vi "Get Selected Text Format.vi"(8 "Error In":errorcluster, 11 "Text Formatting in":T5 {"Font Size" min=6.0 step=1.0}) -> (0 "Error Out":errorcluster, 3 "Text Formatting":T4={"Font"=0, "Text Color"=enum."Unchanged", "Background Color"=enum."Unchanged", "Style"=enum."Regular", "Font Size"=6.0, "Alignment"=enum."Left"} {"Font Size" min=6.0 step=1.0; "Font" items=["Adobe Devanagari", "Agency FB", "Algerian", "Arial", "Arial Black", "Arial Narrow", "Arial Rounded MT Bold", "Bahnschrift", "Bahnschrift Condensed", "Bahnschrift Light", "Bahnschrift Light Condensed", "Bahnschrift Light SemiCondensed", "Bahnschrift SemiBold", "Bahnschrift SemiBold Condensed", "Bahnschrift SemiBold SemiConden", "Bahnschrift SemiCondensed", "Bahnschrift SemiLight", "Bahnschrift SemiLight Condensed", "Bahnschrift SemiLight SemiConde", "Barlow Condensed", "Barlow Condensed Black", "Barlow Condensed ExtraBold", "Barlow Condensed ExtraLight", "Barlow Condensed Light", "Barlow Condensed Medium", "Barlow Condensed SemiBold", "Barlow Condensed Thin", "Baskerville Old Face", "Bauhaus 93", "Bell MT", "Berlin Sans FB", "Berlin Sans FB Demi", "Bernard MT Condensed", "Blackadder ITC", "Bodoni MT", "Bodoni MT Black", "Bodoni MT Condensed", "Bodoni MT Poster Compressed", "Book Antiqua", "Bookman Old Style", "Bookshelf Symbol 7", "Bradley Hand ITC", "Britannic Bold", "Broadway", "Brush Script MT", "Calibri", "Calibri Light", "Californian FB", "Calisto MT", "Cambria", "Cambria Math", "Candara", "Candara Light", "Cascadia Code", "Cascadia Code ExtraLight", "Cascadia Code Light", "Cascadia Code SemiBold", "Cascadia Code SemiLight", "Cascadia Mono", "Cascadia Mono ExtraLight", "Cascadia Mono Light", "Cascadia Mono SemiBold", "Cascadia Mono SemiLight", "Castellar", "Caveat", "Centaur", "Century", "Century Gothic", "Century Schoolbook", "Chiller", "Colonna MT", "Comic Sans MS", "Consolas", "Constantia", "Cooper Black", "Copperplate Gothic Bold", "Copperplate Gothic Light", "Corbel", "Corbel Light", "Cormorant Infant", "Cormorant Infant Light", "Cormorant Infant Medium", "Cormorant Infant SemiBold", "Courier New", "Curlz MT", "Dosis", "Dubai", "Dubai Light", "Dubai Medium", "Ebrima", "Edwardian Script ITC", "Elephant", "Engravers MT", "Eras Bold ITC", "Eras Demi ITC", "Eras Light ITC", "Eras Medium ITC", "Euclid", "Euclid Extra", "Euclid Fraktur", "Euclid Math One", "Euclid Math Two", "Euclid Symbol", "Felix Titling", "Fences", "Footlight MT Light", "Forte", "Franklin Gothic Book", "Franklin Gothic Demi", "Franklin Gothic Demi Cond", "Franklin Gothic Heavy", "Franklin Gothic Medium", "Franklin Gothic Medium Cond", "Freestyle Script", "French Script MT", "Gabriola", "Gadugi", "Garamond", "Georgia", "Gigi", "Gill Sans MT", "Gill Sans MT Condensed", "Gill Sans MT Ext Condensed Bold", "Gill Sans Ultra Bold", "Gill Sans Ultra Bold Condensed", "Gloucester MT Extra Condensed", "Goudy Old Style", "Goudy Stout", "Haettenschweiler", "Harlow Solid Italic", "Harrington", "High Tower Text", "HoloLens MDL2 Assets", "HYSWLongFangSong", "Impact", "Imprint MT Shadow", "Informal Roman", "Ink Free", "Javanese Text", "Jokerman", "Juice ITC", "Kristen ITC", "Kunstler Script", "Lato", "Lato Black", "Lato Hairline", "Lato Light", "Leelawadee", "Leelawadee UI", "Leelawadee UI Semilight", "Lucida Bright", "Lucida Calligraphy", "Lucida Console", "Lucida Fax", "Lucida Handwriting", "Lucida Sans", "Lucida Sans Typewriter", "Lucida Sans Unicode", "Magneto", "Maiandra GD", "Malgun Gothic", "Malgun Gothic Semilight", "Marlett", "Matura MT Script Capitals", "Microsoft Himalaya", "Microsoft JhengHei", "Microsoft JhengHei Light", "Microsoft JhengHei UI", "Microsoft JhengHei UI Light", "Microsoft New Tai Lue", "Microsoft PhagsPa", "Microsoft Sans Serif", "Microsoft Tai Le", "Microsoft Uighur", "Microsoft YaHei", "Microsoft YaHei Light", "Microsoft YaHei UI", "Microsoft YaHei UI Light", "Microsoft Yi Baiti", "MingLiU-ExtB", "MingLiU_HKSCS-ExtB", "Mistral", "Modern No. 20", "Mongolian Baiti", "Monotype Corsiva", "Montserrat", "Montserrat Black", "Montserrat ExtraBold", "Montserrat ExtraLight", "Montserrat Light", "Montserrat Medium", "Montserrat SemiBold", "Montserrat Thin", "MS Gothic", "MS Outlook", "MS PGothic", "MS Reference Sans Serif", "MS Reference Specialty", "MS UI Gothic", "MT Extra", "MT Extra Tiger", "MV Boli", "Myanmar Text", "Niagara Engraved", "Niagara Solid", "Nirmala UI", "Nirmala UI Semilight", "Noto Sans", "Noto Serif", "NSimSun", "OCR A Extended", "Old English Text MT", "Onyx", "Open Sans", "Open Sans ExtraBold", "Open Sans Light", "Open Sans SemiBold", "Origin", "Oswald", "Oswald ExtraLight", "Oswald Light", "Oswald Medium", "Oswald SemiBold", "Palace Script MT", "Palatino Linotype", "Papyrus", "Parchment", "Perpetua", "Perpetua Titling MT", "Playbill", "PMingLiU-ExtB", "Poor Richard", "Pristina", "Rage Italic", "Raleway", "Raleway Black", "Raleway ExtraBold", "Raleway ExtraLight", "Raleway Light", "Raleway Medium", "Raleway SemiBold", "Raleway Thin", "Ravie", "Roboto", "Roboto Black", "Roboto Condensed", "Roboto Condensed Light", "Roboto Light", "Roboto Medium", "Roboto Slab", "Roboto Slab Black", "Roboto Slab Light", "Roboto Slab Medium", "Roboto Slab Thin", "Roboto Thin", "Rockwell", "Rockwell Condensed", "Rockwell Extra Bold", "Script MT Bold", "Segoe MDL2 Assets", "Segoe Print", "Segoe Script", "Segoe UI", "Segoe UI Black", "Segoe UI Emoji", "Segoe UI Historic", "Segoe UI Light", "Segoe UI Semibold", "Segoe UI Semilight", "Segoe UI Symbol", "Showcard Gothic", "SimSun", "SimSun-ExtB", "SimSun-ExtG", "Sitka Banner", "Sitka Display", "Sitka Heading", "Sitka Small", "Sitka Subheading", "Sitka Text", "Snap ITC", "Source Code Pro", "Source Code Pro Black", "Source Code Pro ExtraLight", "Source Code Pro Light", "Source Code Pro Semibold", "Source Sans Pro", "Source Sans Pro Black", "Source Sans Pro ExtraLight", "Source Sans Pro Light", "Source Sans Pro SemiBold", "Stencil", "Sylfaen", "Symbol", "Symbol Tiger", "Symbol Tiger Expert", "Tahoma", "Tempus Sans ITC", "Tiger", "Tiger Expert", "Times New Roman", "Trebuchet MS", "Tw Cen MT", "Tw Cen MT Condensed", "Tw Cen MT Condensed Extra Bold", "Univers-CondBoldOblique", "Univers-Condensed", "Univers-CondensedBold", "UniversCond", "UniversCondBold", "UniversCondLight", "UniversCondLightOblique", "UniversCondOblique", "Verdana", "Viner Hand ITC", "Vivaldi", "Vladimir Script", "Webdings", "Wide Latin", "Wingdings", "Wingdings 2", "Wingdings 3", "Yu Gothic", "Yu Gothic Light", "Yu Gothic Medium", "Yu Gothic UI", "Yu Gothic UI Light", "Yu Gothic UI Semibold", "Yu Gothic UI Semilight", "Zilla Slab", "Zilla Slab Light", "Zilla Slab Medium", "Zilla Slab SemiBold", "ZWAdobeF"]})   [LabVIEW 2021, in "Notebook.lvlib"]
uses:
  Notebook.lvlib
  Rich Text Box/Text Formatting.ctl
  Rich Text Box/Text Colors.ctl
  Rich Text Box/Text Style.ctl
  Rich Text Box/Text Alignment.ctl
  Rich Text Box/Rich Text Box.lvlib
panel:
  # "see the License on the block diagram (Ctrl+E or Window:Show Block Diagram)"
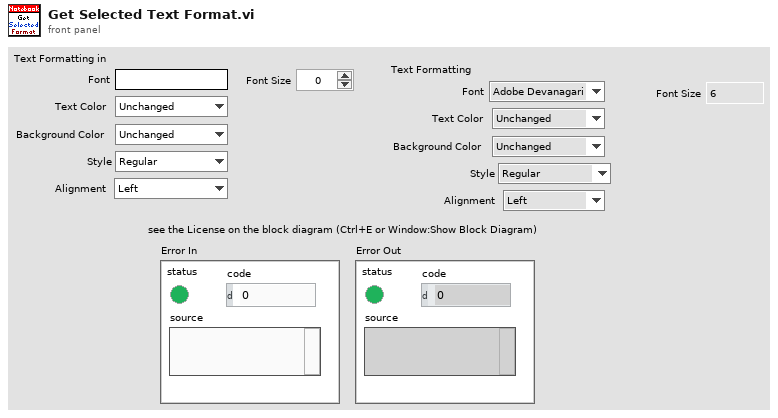
[diagram p1: front panel]
types:
  T1 = typedef "Rich Text Box.lvlib/Text Colors.ctl" = enum16{"Unchanged", "Black", "Blue", "Cyan", "Maroon", "Gray", "Violet", "Green", "Light Green", "Orange", "Yellow", "Magenta", "Red", "White"}
  T2 = typedef "Rich Text Box.lvlib/Text Style.ctl" = enum16{"Regular", "Bold", "Italic", "Underline", "Strikeout"}
  T3 = typedef "Rich Text Box.lvlib/Text Alignment.ctl" = enum16{"Left", "Right", "Center"}
  T4 = cluster{"Font":u16, "Text Color":T1, "Background Color":T1, "Style":T2, "Font Size":dbl, "Alignment":T3}
  T5 = typedef "Rich Text Box.lvlib/Text Formatting.ctl" = cluster{"Font":string, "Text Color":T1, "Background Color":T1, "Style":T2, "Font Size":dbl, "Alignment":T3}
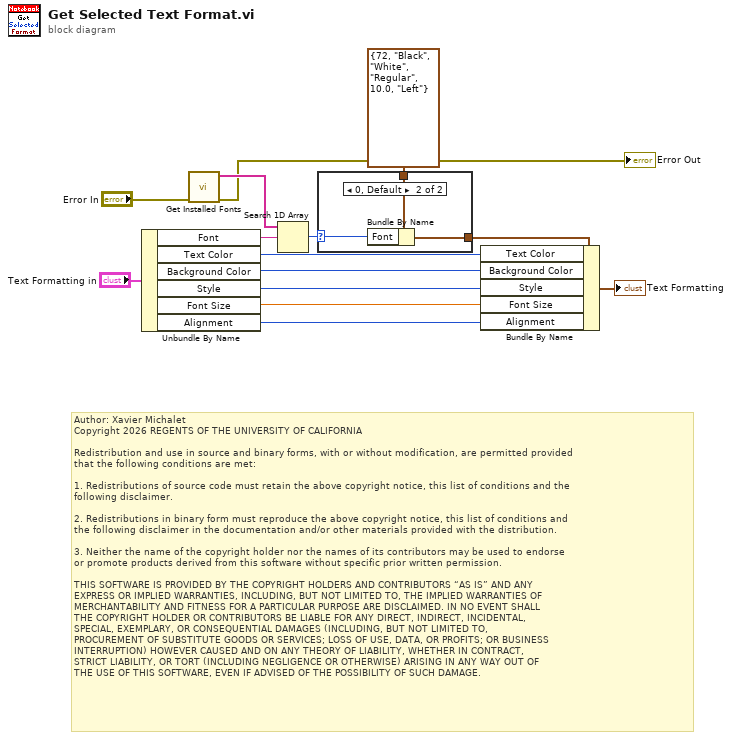
[diagram p0: block diagram]
diagram:
  # "Author: Xavier Michalet\nCopyright 2026 REGENTS OF THE UNIVERSITY OF CALIFORNIA\n\nRedistribution and use in source and binary forms, with or without modification, are permitted provided\nthat the following conditions are met:\n\n1. Redistributions of source code must retain the above copyright notice, this list of conditions and the\nfollowing disclaimer.\n\n2. Redistributions in binary form must reproduce the above copyright notice, this list of conditions and\nthe following disclaimer in the documentation and/or other materials provided with the distribution.\n\n3. Neither the name of the copyright holder nor the names of its contributors may be used to endorse \nor promote products derived from this software without specific prior written permission.\n\nTHIS SOFTWARE IS PROVIDED BY THE COPYRIGHT HOLDERS AND CONTRIBUTORS “AS IS” AND ANY \nEXPRESS OR IMPLIED WARRANTIES, INCLUDING, BUT NOT LIMITED TO, THE IMPLIED WARRANTIES OF\nMERCHANTABILITY AND FITNESS FOR A PARTICULAR PURPOSE ARE DISCLAIMED. IN NO EVENT SHALL\nTHE COPYRIGHT HOLDER OR CONTRIBUTORS BE LIABLE FOR ANY DIRECT, INDIRECT, INCIDENTAL, \nSPECIAL, EXEMPLARY, OR CONSEQUENTIAL DAMAGES (INCLUDING, BUT NOT LIMITED TO, \nPROCUREMENT OF SUBSTITUTE GOODS OR SERVICES; LOSS OF USE, DATA, OR PROFITS; OR BUSINESS\nINTERRUPTION) HOWEVER CAUSED AND ON ANY THEORY OF LIABILITY, WHETHER IN CONTRACT, \nSTRICT LIABILITY, OR TORT (INCLUDING NEGLIGENCE OR OTHERWISE) ARISING IN ANY WAY OUT OF\nTHE USE OF THIS SOFTWARE, EVEN IF ADVISED OF THE POSSIBILITY OF SUCH DAMAGE."
  n1 = Unbundle By Name("Text Formatting in") -> ("Font"=w13:string, "Text Color"=w6:T1, "Background Color"=w5:T1, "Style"=w4:T2, "Font Size"=w3:dbl, "Alignment"=w2:T3)
  n2 = call "Get Installed Fonts.vi"("Error In"="Error In") -> ("Error Out"=→"Error Out":errorcluster, "Installed Fonts"=w11:string[])  [unwired: 8 in, 1 out]
  n3 = Search 1D Array(1D array=w11, element=w13) -> (index of element=w9:i32)  [unwired: 1 in]
  n4 = case shown="0, Default" w9 {
    selector: w9 -> [_ w17]
    tunnel: T4 {"Font"=72, "Text Color"=enum."Black", "Background Color"=enum."White", "Style"=enum."Regular", "Font Size"=10.0, "Alignment"=enum."Left"} ("Text Formatting") -> [w15 w18]
    tunnel: [w15 w16] -> w8
    frame -1 {
    }
    frame 0, Default {
      n5 = Bundle By Name(cluster=w18, "Font"=w17) -> (w16:T4)
    }
  }
  n6 = Bundle By Name(cluster=w8, "Text Color"=w6, "Background Color"=w5, "Style"=w4, "Font Size"=w3, "Alignment"=w2) -> (→"Text Formatting":T4)
